vi "testChem2.vi"() -> ()   [LabVIEW 2012]
uses:
  <vilib>/Utility/file.llb/Read From Spreadsheet File (string).vi
  <userlib>/ImageProcessing/InitCamera_NTSC.vi
  <userlib>/ImageProcessing/FilterGreenPlane.vi
  <userlib>/ImageProcessing/FilterRedPlane.vi
panel:
  out "Array":string[](array[string])
  out "Element":string[](array[string])
  out "indexsWhereTrue":i32[](array[numeric])
  out "Min":dbl[](array[numeric])
  out "Max":dbl[](array[numeric])
  out "x+y":dbl[](array[numeric])
  out "S4":dbl[](array[numeric])
  out "S3":dbl[](array[numeric])
  out "S2":dbl[](array[numeric])
  out "S1":dbl[](array[numeric])
  in  "Path":path
  out "Periodic":string[][](array[string])
  out "image 2":picture
  out "Ra4":dbl
  out "Ra3":dbl
  out "Ra2":dbl
  out "Ra1":dbl
  out "A4":dbl
  out "A3":dbl
  out "A2":dbl
  out "A1":dbl
  out "a4":dbl
  out "a3":dbl
  out "a2":dbl
  out "a1":dbl
  out "Centroid 4":cluster{"X":dbl, "Y":dbl}
  out "Centroid 3":cluster{"X":dbl, "Y":dbl}
  out "Centroid 2":cluster{"X":dbl, "Y":dbl}
  out "Centroid":cluster{"X":dbl, "Y":dbl}
  out "initialized array 2":dbl[][](array[numeric])
  out "image":picture
  in  "Stop":bool
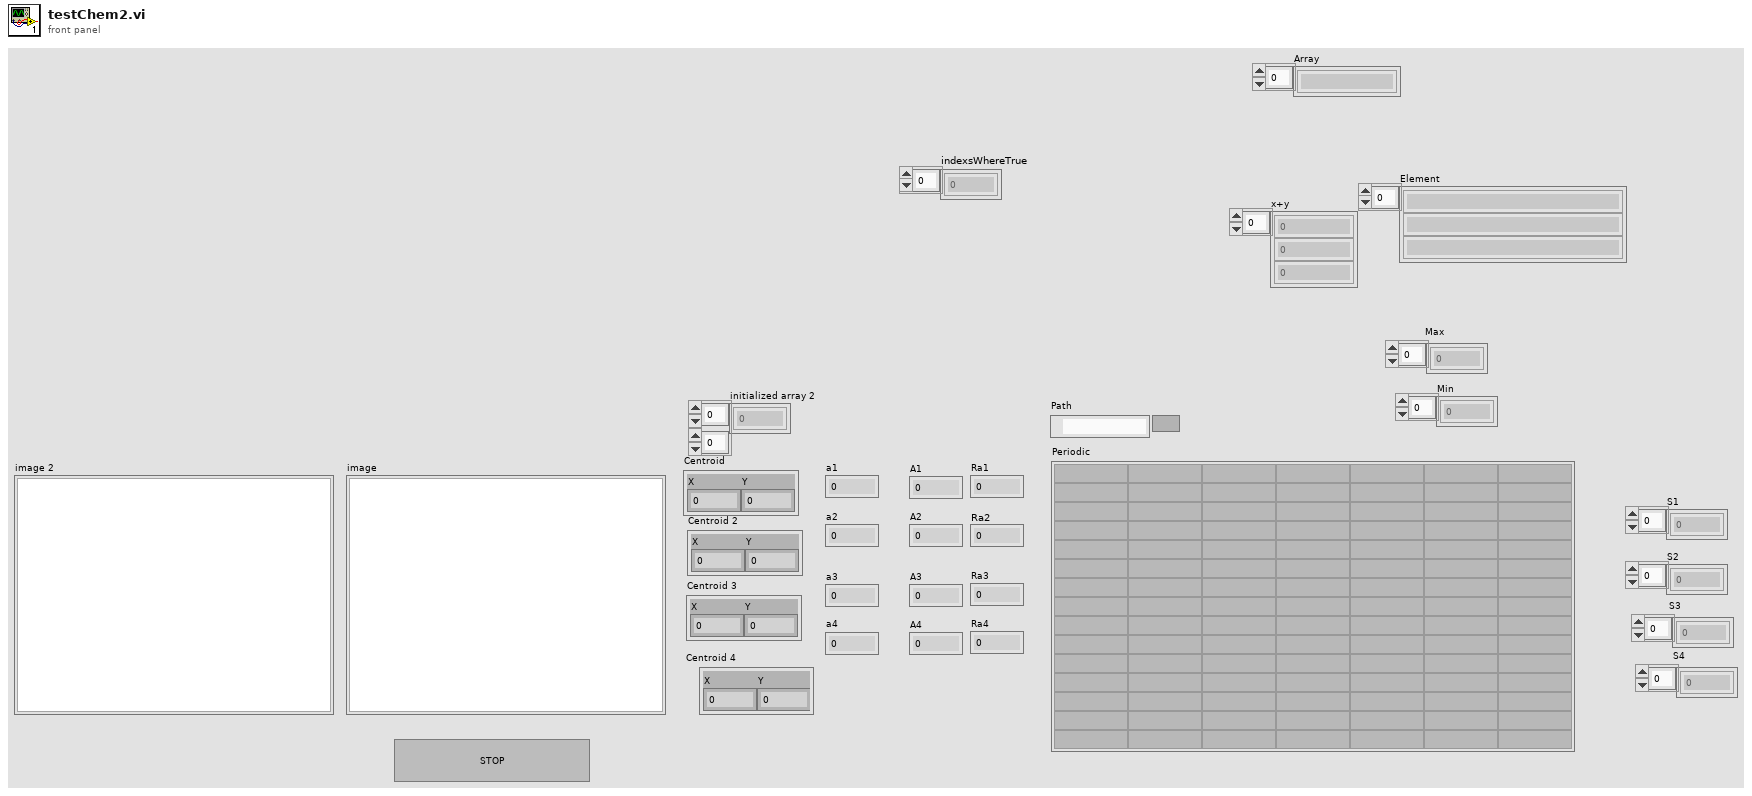
[diagram p1: front panel]
types:
  T1 = typedef "QT_Ref.ctl" = refnum<k1>
  T2 = cluster{"Width":u16, "Style":enum32{"Solid", "Dash", "Dot", "DashDot", "DashDotDot"}}
  T3 = typedef "QT_Image.ctl" = cluster{"Width":i32, "Height":i32, "Depth":i32, "data":u8[], "Compressed data":u8[], "Color table":u32[], "Duration":i32, "Options":i32, "Timestamp":i32, "ID":i32, "Reserved":i32, "Dialogs":u32}
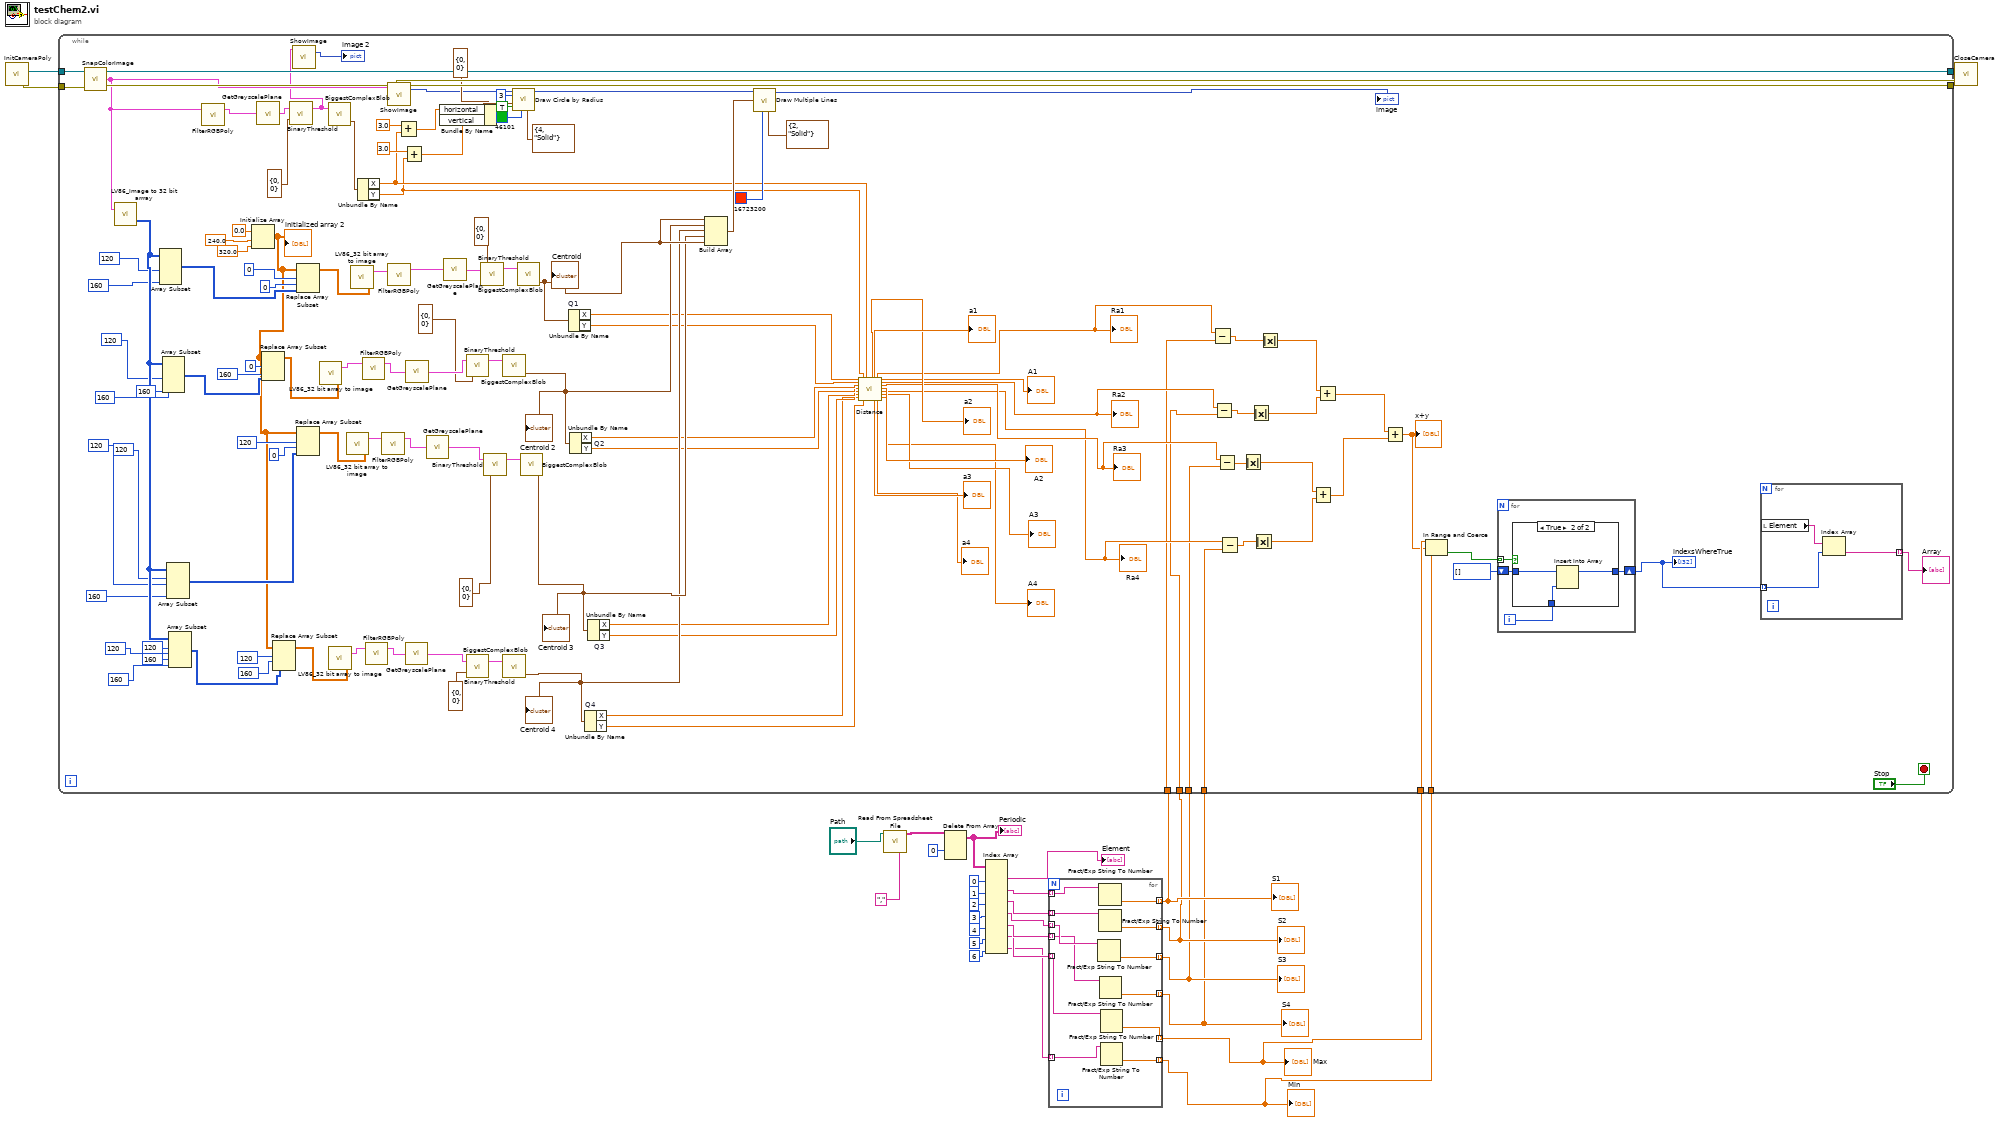
[diagram p0: block diagram]
diagram:
  n1 = call-poly <userlib>:"InitCameraPoly.vi"() -> ("error out"=w26:errorcluster, "QT Ref Out"=w27:T1)  [unwired: 2 in]
  n2 = call-poly <vilib>:"Read From Spreadsheet File.vi"("delimiter (\\t)"="," ("delimiter (\\t)"), "file path (dialog if empty)"="Path") -> ("all rows"=w25:string[][])  [unwired: 5 in, 4 out]
  n3 = Delete From Array(array=w25, index (row)=0) -> (array with subset deleted=w2:string[][])  [unwired: 2 in, 1 out]
  "Periodic" <- w2
  n4 = Index Array(array=w2, index (col) #1=0 ("disabled index (col)"), index (col) #2=1 ("index (col)"), index (col) #3=2 ("index (col)"), index (col) #4=3 ("index (col)"), index (col) #5=4 ("index (col)"), index (col) #6=5 ("index (col)"), index (col) #7=6 ("index (col)")) -> (element #1=→"Element":string[], element #2=w18:string[], element #3=w17:string[], element #4=w14:string[], element #5=w13:string[], element #6=w6:string[], element #7=w5:string[])  [unwired: 7 in]
  n5 = for {
    tunnel: w18 -> [w41] mode=indexing
    tunnel: w17 -> [w40] mode=indexing
    tunnel: [w39] -> w12 mode=indexing
    tunnel: [w38] -> w11 mode=indexing
    tunnel: [w37] -> w10 mode=indexing
    tunnel: w14 -> [w36] mode=indexing
    tunnel: w13 -> [w35] mode=indexing
    tunnel: [w34] -> w9 mode=indexing
    tunnel: w6 -> [w33] mode=indexing
    tunnel: w5 -> [w32] mode=indexing
    tunnel: [w31] -> w4 mode=indexing
    tunnel: [w30] -> w3 mode=indexing
    n6 = Fract/Exp String To Number(string=w36) -> (number=w37:dbl)  [unwired: 3 in, 1 out]
    n7 = Fract/Exp String To Number(string=w41) -> (number=w39:dbl)  [unwired: 3 in, 1 out]
    n8 = Fract/Exp String To Number(string=w40) -> (number=w38:dbl)  [unwired: 3 in, 1 out]
    n9 = Fract/Exp String To Number(string=w35) -> (number=w34:dbl)  [unwired: 3 in, 1 out]
    n10 = Fract/Exp String To Number(string=w33) -> (number=w31:dbl)  [unwired: 3 in, 1 out]
    n11 = Fract/Exp String To Number(string=w32) -> (number=w30:dbl)  [unwired: 3 in, 1 out]
  }
  "S1" <- w12
  "S2" <- w11
  "S3" <- w10
  "S4" <- w9
  "Max" <- w4
  "Min" <- w3
  n12 = while {
    tunnel: w26 -> [w169]
    tunnel: w27 -> [w168]
    tunnel: [w167] -> w28
    tunnel: [w166] -> w29
    tunnel: w12 -> [w62]
    tunnel: w11 -> [w61]
    tunnel: w10 -> [w60]
    tunnel: w9 -> [w59]
    tunnel: w4 -> [w48]
    tunnel: w3 -> [w47]
    stop <- "Stop" stop-if-true
    n13 = call <userlib>:"SnapColorImage.vi"("error in (no error)"=w169, "QT Ref In"=w168) -> ("error out"=w167:errorcluster, "Image Out"=w100:T3, "QT Ref Out"=w166:T1)  [unwired: 1 in]
    n14 = call <userlib>:"LV86_Image to 32 bit arrray.vi"("Image In"=w100) -> ("Intensity Graph"=w164:u32[][])  [unwired: 1 in, 1 out]
    n15 = Array Subset(array=w164, length (row)=120 ("length"), length (col)=160 ("length")) -> (w140:u32[][])  [unwired: 2 in]
    n16 = Array Subset(array=w164, length (row)=120 ("length"), index (col)=160 ("index"), length (col)=160 ("length")) -> (w151:u32[][])  [unwired: 1 in]
    n17 = Array Subset(array=w164, index (row)=120 ("index"), length (row)=120 ("length"), length (col)=160 ("length")) -> (w134:u32[][])  [unwired: 1 in]
    n18 = Array Subset(array=w164, index (row)=120 ("index"), length (row)=120 ("length"), index (col)=160 ("index"), length (col)=160 ("length")) -> (w131:u32[][])
    n19 = call-poly <userlib>:"FilterRGBPoly.vi"("Image in"=w100) -> ("Image out"=w103:T3)  [unwired: 1 in, 1 out]
    n20 = Initialize Array(0.0 ("element"), 240.0 ("element"), 320.0 ("element")) -> (w130:dbl[][])
    "initialized array 2" <- w130
    n21 = call <userlib>:"GetGreyscalePlane.vi"("Image In"=w103) -> ("Greyscale  Out"=w87:T3)
    n22 = Replace Array Subset(array=w130, new element=w151, index (row)=0, index (col)=160 ("index (row)")) -> (w150:dbl[][])
    n23 = Replace Array Subset(array=w130, new element=w131, index (row)=120, index (col)=160 ("index (row)")) -> (w128:dbl[][])
    n24 = call <userlib>:"BinaryThreshold.vi"("threshold"=cluster{u8, u8} {0, 0}, "Image In"=w87) -> ("Image Out"=w85:T3)  [unwired: 1 in]
    n25 = call <userlib>:"ShowImage.vi"("Image"=w85) -> ("image"=→"image 2":picture)  [unwired: 2 in, 1 out]
    n26 = Replace Array Subset(array=w130, new element=w140, index (row)=0, index (col)=0 ("index (row)")) -> (w139:dbl[][])
    n27 = Replace Array Subset(array=w130, new element=w134, index (row)=120, index (col)=0 ("index (row)")) -> (w129:dbl[][])
    n28 = call <userlib>:"LV86_32 bit array to image.vi"("Intensity Graph"=w150) -> ("Image Out"=w127:T3)  [unwired: 2 in]
    n29 = call <userlib>:"BiggestComplexBlob.vi"("Image in"=w85) -> ("Centroid"=w101:cluster{"X":dbl, "Y":dbl})  [unwired: 1 in, 2 out]
    n30 = call <userlib>:"LV86_32 bit array to image.vi"("Intensity Graph"=w128) -> ("Image Out"=w125:T3)  [unwired: 2 in]
    n31 = call <userlib>:"LV86_32 bit array to image.vi"("Intensity Graph"=w129) -> ("Image Out"=w126:T3)  [unwired: 2 in]
    n32 = call <userlib>:"LV86_32 bit array to image.vi"("Intensity Graph"=w139) -> ("Image Out"=w138:T3)  [unwired: 2 in]
    n33 = Unbundle By Name(w101) -> ("X"=w84:dbl, "Y"=w83:dbl)
    n34 = call-poly <userlib>:"FilterRGBPoly.vi"("Image in"=w127) -> ("Image out"=w124:T3)  [unwired: 1 in, 1 out]
    n35 = call-poly <userlib>:"FilterRGBPoly.vi"("Image in"=w125) -> ("Image out"=w122:T3)  [unwired: 1 in, 1 out]
    n36 = call-poly <userlib>:"FilterRGBPoly.vi"("Image in"=w126) -> ("Image out"=w123:T3)  [unwired: 1 in, 1 out]
    n37 = call <userlib>:"ShowImage.vi"("Image"=w100) -> ("image"=w88:picture)  [unwired: 2 in, 1 out]
    n38 = call-poly <userlib>:"FilterRGBPoly.vi"("Image in"=w138) -> ("Image out"=w137:T3)  [unwired: 1 in, 1 out]
    n39 = Add(x=3.0, y=w84) -> (x+y=w94:dbl)
    n40 = Add(x=3.0, y=w83) -> (x+y=w93:dbl)
    n41 = call <userlib>:"GetGreyscalePlane.vi"("Image In"=w122) -> ("Greyscale  Out"=w116:T3)
    n42 = call <userlib>:"GetGreyscalePlane.vi"("Image In"=w124) -> ("Greyscale  Out"=w118:T3)
    n43 = call <userlib>:"GetGreyscalePlane.vi"("Image In"=w123) -> ("Greyscale  Out"=w117:T3)
    n44 = Bundle By Name(cluster=cluster{"horizontal":i16, "vertical":i16} {"horizontal"=0, "vertical"=0} ("pixel center"), "horizontal"=w94, "vertical"=w93) -> (w98:cluster{"horizontal":i16, "vertical":i16})
    n45 = call <userlib>:"GetGreyscalePlane.vi"("Image In"=w137) -> ("Greyscale  Out"=w136:T3)
    n46 = call <userlib>:"BinaryThreshold.vi"("threshold"=cluster{u8, u8} {0, 0}, "Image In"=w118) -> ("Image Out"=w121:T3)  [unwired: 1 in]
    n47 = call <userlib>:"BinaryThreshold.vi"("threshold"=cluster{u8, u8} {0, 0}, "Image In"=w116) -> ("Image Out"=w119:T3)  [unwired: 1 in]
    n48 = call <userlib>:"BinaryThreshold.vi"("threshold"=cluster{u8, u8} {0, 0}, "Image In"=w136) -> ("Image Out"=w135:T3)  [unwired: 1 in]
    n49 = call <userlib>:"BinaryThreshold.vi"("threshold"=cluster{u8, u8} {0, 0}, "Image In"=w117) -> ("Image Out"=w120:T3)  [unwired: 1 in]
    n50 = call <userlib>:"BiggestComplexBlob.vi"("Image in"=w121) -> ("Centroid"=w106:cluster{"X":dbl, "Y":dbl})  [unwired: 1 in, 2 out]
    "Centroid 2" <- w106
    n51 = call <userlib>:"BiggestComplexBlob.vi"("Image in"=w119) -> ("Centroid"=w104:cluster{"X":dbl, "Y":dbl})  [unwired: 1 in, 2 out]
    "Centroid 4" <- w104
    n52 = call <vilib>:"Draw Circle by Radius.vi"("pen"=T2 {"Width"=4, "Style"=enum."Solid"}, "color(black)"=u32 46101, "fill?(F)"=TRUE, "pixel center"=w98, "radius"=i16 3, "picture"=w88) -> ("new picture"=w99:picture)  [unwired: 5 in]
    n53 = call <userlib>:"BiggestComplexBlob.vi"("Image in"=w135) -> ("Centroid"=w107:cluster{"X":dbl, "Y":dbl})  [unwired: 1 in, 2 out]
    "Centroid" <- w107
    n54 = call <userlib>:"BiggestComplexBlob.vi"("Image in"=w120) -> ("Centroid"=w105:cluster{"X":dbl, "Y":dbl})  [unwired: 1 in, 2 out]
    "Centroid 3" <- w105
    n55 = Unbundle By Name "Q1"(w107) -> ("X"=w82:dbl, "Y"=w81:dbl)
    n56 = Unbundle By Name "Q2"(w106) -> ("X"=w80:dbl, "Y"=w79:dbl)
    n57 = Unbundle By Name "Q4"(w104) -> ("X"=w76:dbl, "Y"=w75:dbl)
    n58 = Unbundle By Name "Q3"(w105) -> ("X"=w78:dbl, "Y"=w77:dbl)
    n59 = Build Array(w107, w106, w104, w105, w107) -> (w114:cluster{"X":dbl, "Y":dbl}[])
    n60 = call <vilib>:"Draw Multiple Lines.vi"("picture"=w99, "line endpoints"=w114, "color(black)"=u32 16723200, "pen"=T2 {"Width"=2, "Style"=enum."Solid"}) -> ("new picture"=→"image":picture)  [unwired: 5 in]
    n61 = call "Distance.vi"("X1"=w82, "Y1"=w81, "X2"=w80, "Y2"=w79, "X3"=w78, "Y3"=w77, "x4"=w76, "Y"=w83, "Y4"=w75, "X"=w84) -> ("a2"=→"a2":dbl, "a1"=→"a1":dbl, "a3"=→"a3":dbl, "Ra1"=w66:dbl, "a4"=→"a4":dbl, "A1"=→"A1":dbl, "Ra2"=w65:dbl, "Ra3"=w64:dbl, "A2"=→"A2":dbl, "Ra4"=w63:dbl, "A3"=→"A3":dbl, "A4"=→"A4":dbl)  [unwired: 6 in]
    "Ra1" <- w66
    "Ra2" <- w65
    "Ra3" <- w64
    "Ra4" <- w63
    n62 = Subtract(x=w66, y=w62) -> (x-y=w58:dbl[])
    n63 = Subtract(x=w65, y=w61) -> (x-y=w57:dbl[])
    n64 = Subtract(x=w64, y=w60) -> (x-y=w56:dbl[])
    n65 = Subtract(x=w63, y=w59) -> (x-y=w55:dbl[])
    n66 = Absolute Value(x=w56) -> (abs(x)=w52:dbl[])
    n67 = Absolute Value(x=w57) -> (abs(x)=w53:dbl[])
    n68 = Absolute Value(x=w55) -> (abs(x)=w51:dbl[])
    n69 = Absolute Value(x=w58) -> (abs(x)=w54:dbl[])
    n70 = Add(x=w52, y=w51) -> (x+y=w49:dbl[])
    n71 = Add(x=w54, y=w53) -> (x+y=w50:dbl[])
    n72 = Add(x=w50, y=w49) -> (x+y=w45:dbl[])
    "x+y" <- w45
    n73 = In Range and Coerce(upper limit=w48, x=w45, lower limit=w47) -> (In Range?=w46:bool[])  [unwired: 1 out]
    n74 = for {
      tunnel: w46 -> [w176] mode=indexing
      shift-right: [w174] -> w43
      shift-left: i32[] [] -> [w173]
      i -> [w175]
      n75 = case shown="True" w176 {
        tunnel: w175 -> [_ w180]
        tunnel: [w177 w179] -> w174
        tunnel: w173 -> [w177 w178]
        frame False {
        }
        frame True {
          n76 = Insert Into Array(array=w178, new element=w180) -> (w179:i32[])  [unwired: 1 in]
        }
      }
    }
    "indexsWhereTrue" <- w43
    n77 = for {
      tunnel: w43 -> [w172] mode=indexing
      tunnel: [w170] -> w42 mode=indexing
      n78 = local read "Element"() -> (w171:string[])
      n79 = Index Array(array=w171, index=w172) -> (element=w170:string)
    }
    "Array" <- w42
  }
  n80 = call <userlib>:"CloseCamera.vi"("error in (no error)"=w28, "QT Ref In"=w29) -> ()  [unwired: 1 in, 1 out]
